vi "CData Flatten String.vi"   [LabVIEW 2010]
uses:
  NXTFlattenXNode/CData Flatten XNode.xnode
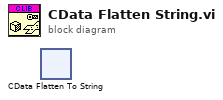
[diagram p0: block diagram]
diagram:
  n1 = xnode "CData Flatten To String"() -> ()  [unwired: 2 in, 2 out]
